vi "Get_Sweep_Wavelength.vi"(8 "error in (no error)":errorcluster, 11 ".NET Reference in":refnum<k24>) -> (0 "error out":errorcluster, 1 "endwave out":dbl, 2 "startwave out":dbl, 3 ".NET Reference out":refnum<k24>)   [LabVIEW 2017]
uses:
  C:/Users/Ssantec_Test/Documents/Instrument_DLL_Sample_Labview_20220902_Ver1.2.2/DLL/x86/InstrumentDLL.dll
  DLL/x86/InstrumentDLL.dll
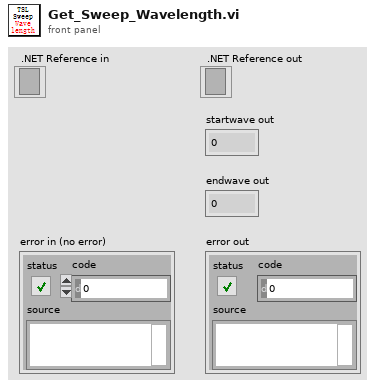
[diagram p1: front panel]
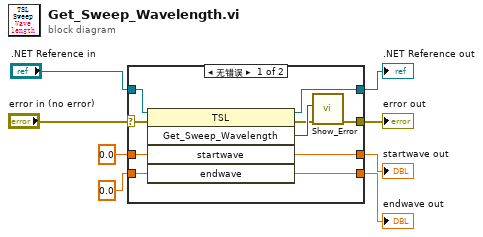
[diagram p0: block diagram]
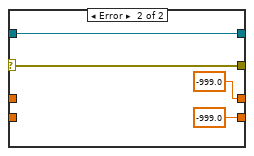
[diagram p2: hidden frame]
diagram:
  n1 = case shown="无错误" "error in (no error)" {
    selector: "error in (no error)" -> [w9 w20]
    tunnel: [w18 -999.0 ("endwave")] -> w8
    tunnel: [w17 -999.0 ("startwave")] -> w7
    tunnel: ".NET Reference in" -> [w16 w19]
    tunnel: [w10 w20] -> w5
    tunnel: [w15 w19] -> w4
    tunnel: 0.0 ("startwave") -> [w14 _]
    tunnel: 0.0 ("endwave") -> [w13 _]
    frame No Error {
      n2 = invoke on="调用节点" class="TSL" method="Get_Sweep_Wavelength"(reference=w16, error in=w9, "startwave"=w14, "endwave"=w13) -> (reference out=w15:refnum<k24>, error out=w11:errorcluster, "Get_Sweep_Wavelength"=w12:i32, "startwave"=w17:dbl, "endwave"=w18:dbl)  [unwired: 1 in]
      n3 = call "Show_Error.vi"("error in (no error)"=w11, "Error"=w12) -> ("error out"=w10:errorcluster)  [unwired: 9 in]
    }
    frame Error {
    }
  }
  "endwave out" <- w8
  "startwave out" <- w7
  "error out" <- w5
  ".NET Reference out" <- w4
